vi "GetIMOrder.vi"(6 "Legacy (f)?":bool, 8 "error in (no error)":errorcluster) -> (0 "error out":errorcluster, 2 "IMOrder":u8)   [LabVIEW 2011]
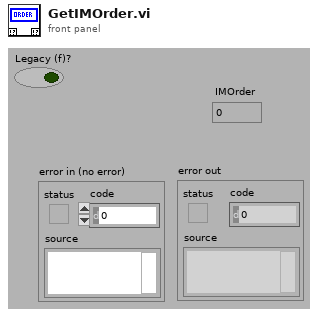
[diagram p1: front panel]
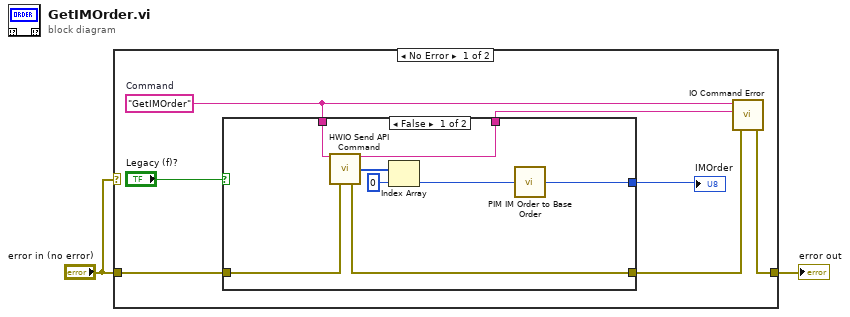
[diagram p0: block diagram]
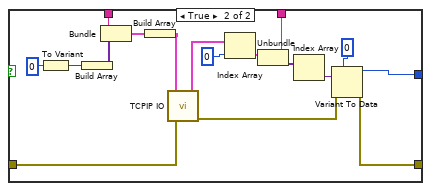
[diagram p2: hidden frame]
diagram:
  n1 = case shown="No Error" "error in (no error)" {
    tunnel: "error in (no error)" -> [w4 w35]
    tunnel: [w8 w35] -> w2
    frame No Error {
      w7 = "GetIMOrder"  # Command
      n2 = case shown="False" "Legacy (f)?" {
        tunnel: [w10 w29] -> w9
        tunnel: w7 -> [w14 w27]
        tunnel: [w15 w26] -> w6
        tunnel: w4 -> [w17 w19]
        tunnel: [w16 w18] -> w3
        frame False {
          n3 = call "HWIO Send API Command.vi"("Action"=w14, "error in (no error)"=w17) -> ("Action out"=w15:string, "Integer out"=w13:i32[], "error out"=w16:errorcluster)  [unwired: 6 in, 5 out]
          n4 = Index Array(array=w13, index=0) -> (element=w11:i32)
          n5 = call "PIM IM Order to Base Order.vi"("IM Order"=w11) -> ("Base Order Index"=w10:u8)
        }
        frame True {
          n6 = To Variant(anything=u8 0) -> (Variant=w34:variant)
          n7 = Build Array(w34) -> (w32:variant[])
          n8 = Bundle("Command"=w27, w32) -> (w31:cluster{"Command":string, variant[]})  [unwired: 1 out]
          n9 = Build Array(w31) -> (w28:cluster{"Command":string, variant[]}[])
          n10 = call "TCPIP IO.vi"("error in (no error)"=w19, "Commands"=w28) -> ("error out"=w20:errorcluster, "Responses"=w25:cluster{string, variant[]}[])  [unwired: 1 in, 3 out]
          n11 = Index Array(array=w25, index=0) -> (element=w24:cluster{string, variant[]})
          n12 = Unbundle(w24) -> (w26:string, w23:variant[])
          n13 = Index Array(array=w23) -> (element=w22:variant)  [unwired: 1 in]
          n14 = Variant To Data(error in=w20, type=u8 0, Variant=w22) -> (data=w29:u8, error out=w18:errorcluster)
        }
      }
      "IMOrder" <- w9
      n15 = call "IO Command Error.vi"("error in (no error)"=w3, "Command Returned (\"\")"=w6, "Command Sent (\"\")"=w7) -> ("error out"=w8:errorcluster)  [unwired: 4 out]
    }
    frame Error {
    }
  }
  "error out" <- w2
